vi "_TangoWriteFloatImageAttribute.vi"(1 "error in":errorcluster, 2 "value":sgl[][](array[numeric]), 3 "attribute name":string, 4 "device name":string) -> (0 "error out":errorcluster)   [LabVIEW 2014, in "tango.lvlib"]
uses:
  tango.lvlib
  Insertors/base/fromFloatImage.vi
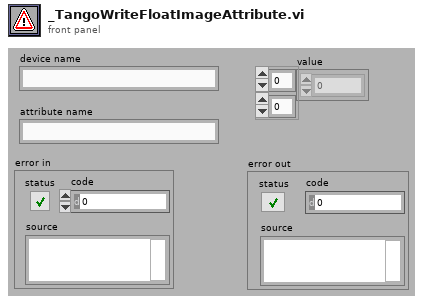
[diagram p1: front panel]
types:
  T1 = typedef "tango.lvlib/_AttributeValue_t.ctl" = cluster{"device name":string, "attribute name":string, "quality value":T2, "quality string":string, "timestamp":dbl, "dim. x":i32, "dim. y":i32, "value":u8[], "error code":i32, "error stack":string[], "data type":T3}
  T2 = typedef "tango.lvlib/_AttributeQuality_t.ctl" = enum16{"VALID", "INVALID", "ALARM", "CHANGING", "UNKNOWN_QUALITY"}
  T3 = typedef "tango.lvlib/_AttributeDataType_t.ctl" = enum16{"STATE_SCA", "STATE_SPE", "STATE_IMG", "STRING_SCA", "STRING_SPE", "STRING_IMG", "BOOL_SCA", "BOOL_SPE", "BOOL_IMG", "UCHAR_SCA", "UCHAR_SPE", "UCHAR_IMG", "SHORT_SCA", "SHORT_SPE", "SHORT_IMG", "USHORT_SCA", "USHORT_SPE", "USHORT_IMG", "LONG_SCA", "LONG_SPE", "LONG_IMG", "ULONG_SCA", "ULONG_SPE", "ULONG_IMG", "LONG64_SCA", "LONG64_SPE", "LONG64_IMG", "ULONG64_SCA", "ULONG64_SPE", "ULONG64_IMG", "FLOAT_SCA", "FLOAT_SPE", "FLOAT_IMG", "DOUBLE_SCA", "DOUBLE_SPE", "DOUBLE_IMG", "UNKNOWN_DATA_TYPE"}
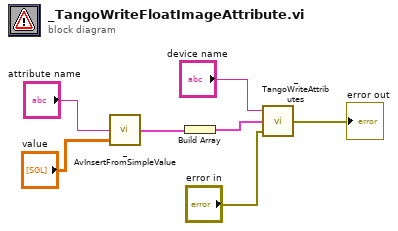
[diagram p0: block diagram]
diagram:
  n1 = call-poly "_AvInsertFromSimpleValue.vi"("value"="value", "attribute name"="attribute name") -> ("attribute value"=w4:T1)  [unwired: 1 in]
  n2 = Build Array(w4) -> (w6:T1[])
  n3 = call "_TangoWriteAttributes.vi"("error in"="error in", "attribute Values"=w6, "device name"="device name") -> ("error out"=→"error out":errorcluster)
